vi "tool go3.vi"(4 "sensor angle":dbl=0.7625468656636853, 5 "assembly angle":dbl=0.7934896104592445, 6 "sensor center":dbl[](array[numeric])=[1019.8477869592303, 797.7567932559023], 7 "assembly center":dbl[](array[numeric])=[988.6776511594305, 1093.1610787780178], 9 "motion":T3={"XYZU "=[], "XY speed"=20.0, "Z speed"=3.0, "U speed"=0.0}, 10 "z offset":T1={"Syringe Z0"=65.0, "assembly thickness"=1.476, "tool height"=9.5, "Gule thickness "=0.1, "Pick Up Tool Z height"=63.541299073279426, "assembly Z offset"=-4.7, "gule distances"=0.6, "Syringe Z height abs"=53.424, "assembly Z height abs"=56.041299073279426, "Syringe Z height rel"=-11.576, "assembly Z height rel"=-2.8, "component  thickness"=1.224}, 11 "controller in":T4={"A3200.lvclass"=refnum, "Ultimus V2.lvclass"=refnum, "NI-DAQ.lvclass"=refnum, "Motion.lvclass"=refnum, "I-O.lvclass"=refnum, "Dispenser.lvclass"=refnum}) -> (2 "z offset out":T1={"Syringe Z0"=65.0, "assembly thickness"=1.476, "tool height"=9.5, "Gule thickness "=0.1, "Pick Up Tool Z height"=63.541299073279426, "assembly Z offset"=-4.7, "gule distances"=0.6, "Syringe Z height abs"=53.424, "assembly Z height abs"=56.041299073279426, "Syringe Z height rel"=-11.576, "assembly Z height rel"=-2.8, "component  thickness"=1.224}, 3 "controller out":T4)   [LabVIEW 2016]
uses:
  Classes/Controller/Motion/A3200 Folder/A3200.lvclass
  D:/Gantry_General/Classes/Controller/Motion/Motion Folder/Motion.lvclass
  Classes/Controller/Dispenser/Ultimus V2 Folder/Ultimus V2.lvclass
  Classes/Controller/I-O/NI-DAQ Folder/NI-DAQ.lvclass
  D:/Gantry_General/Classes/Controller/I-O/I-O Folder/I-O.lvclass
  Classes/Controller/Motion/Motion Folder/Motion.lvclass
  Classes/Controller/I-O/I-O Folder/I-O.lvclass
  Classes/Controller/Dispenser/Dispenser Folder/Dispenser.lvclass
panel:
  in  "run 2":bool
  in  "run":bool
  in  "Tab Control":T2(tab)=enum."motion"
  in  "go to assembly xyzu":bool
  in  "get assembly xyzu":bool
  out "assembly xyzu":dbl[](array[numeric])=[868.8146511594305, 1082.6710787780178, 56.041299073279426, 0.03094274479555914]
  in  "go to assembly center":bool
  in  "get assembly center":bool
  in  "go to tool center":bool
  in  "go to sensor center":bool
  in  "Bellows tool offset":dbl[](array[numeric])=[-119.863, -10.49, 0.0, 0.0]
  in  "get tool center":bool
  in  "tooling center":dbl[](array[numeric])=[1209.998534492856, 792.2969774938225]
  in  "get sensor center":bool
  in  "tooling angle":dbl=0.0876326779785796
  in  "Speed":dbl=30.0
  in  "Delay Time (s)":dbl=10.0
  out "angle":dbl=1.772888683335932
  in  "assembly z":dbl=57.43
  in  "get tooling xyzu":bool
  out "tooling center xyzu":dbl[](array[numeric])=[1090.1355344928559, 781.8069774938225, 0.0, 0.0]
  in  "go to tooling center xyzu":bool
  in  "z go":bool
  out "Sum":dbl[](array[numeric])=[1219.30639899585, 722.8896830877354, 52.864847366341415, 0.003106741190800654] format="%#_8g"
  in  "joystick and camera":bool
  in  "set z height":bool
  out "XYZTheta Out":dbl[](array[numeric])=[1090.1355359956099, 781.8069698988636, 63.541299073279426, 9.091827430758793e-07]
  in  "z to zero":bool
  in  "go to Lower stop":bool
  out "Boolean":bool
  in  "Position":dbl format="%#_13g"
  in  "IO 1":bool
  in  "IO 2":bool
  in  "Values":bool[](array[boolean])=[FALSE, FALSE]
  in  "Indices":i32[](array[numeric])=[0, 20]
  in  "Value":bool
  in  "Channel":i32
  out "Array 2":bool[](array[boolean])
  out "Value 2":bool
  in  "stop":bool
  # "57.53"
  # "57.21"
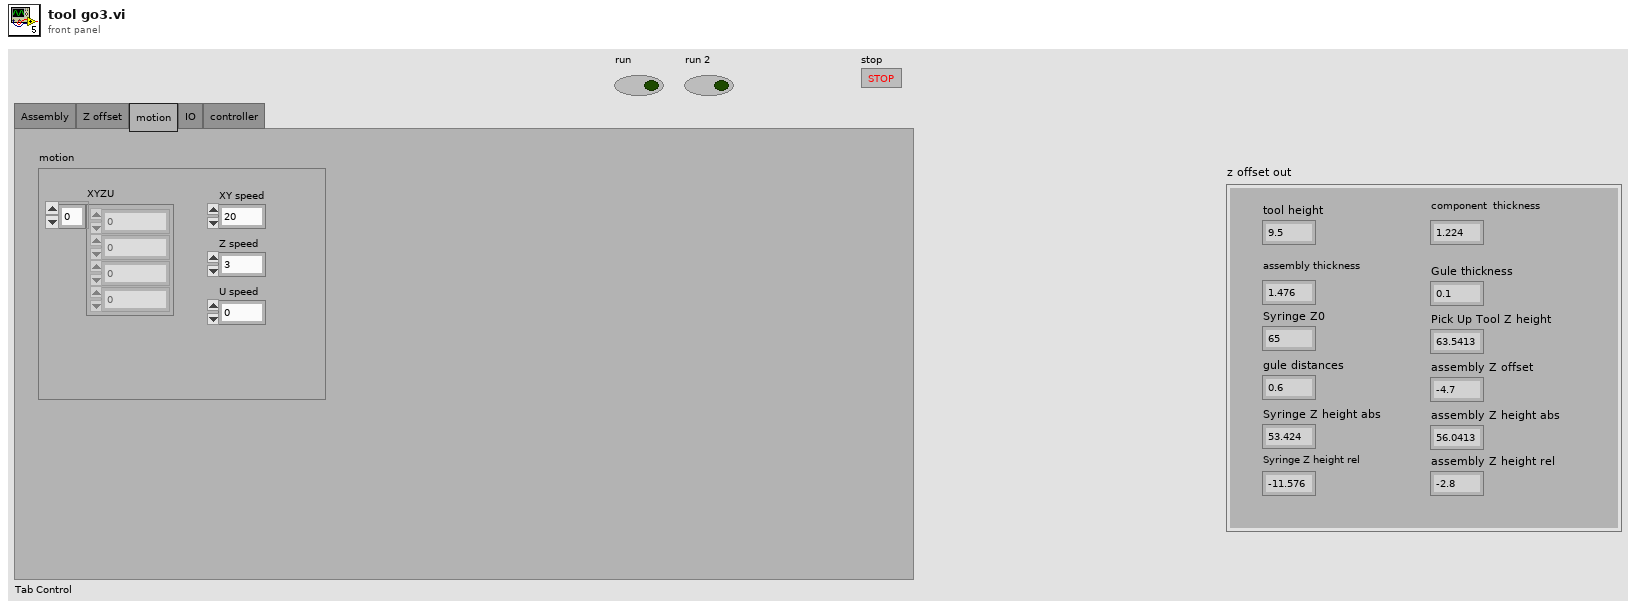
[diagram p1: front panel]
types:
  T1 = cluster{"Syringe Z0":dbl, "assembly thickness":dbl, "tool height":dbl, "Gule thickness ":dbl, "Pick Up Tool Z height":dbl, "assembly Z offset":dbl, "gule distances":dbl, "Syringe Z height abs":dbl, "assembly Z height abs":dbl, "Syringe Z height rel":dbl, "assembly Z height rel":dbl, "component  thickness":dbl}
  T2 = enum32{"Assembly", "Z offset", "motion", "IO", "controller"}
  T3 = cluster{"XYZU ":dbl[], "XY speed":dbl, "Z speed":dbl, "U speed":dbl}
  T4 = cluster{"A3200.lvclass":refnum<class "A3200.lvclass">, "Ultimus V2.lvclass":refnum<class "Ultimus V2.lvclass">, "NI-DAQ.lvclass":refnum<class "NI-DAQ.lvclass">, "Motion.lvclass":refnum<class "Motion.lvclass">, "I-O.lvclass":refnum<class "I-O.lvclass">, "Dispenser.lvclass":refnum<class "Dispenser.lvclass">}
  T5 = cluster{"Bellows tool offset":dbl[], "tooling center":dbl[], "tooling angle ":dbl, "sensor center":dbl[], "sensor angle":dbl, "assembly center":dbl[], "assembly angle":dbl}
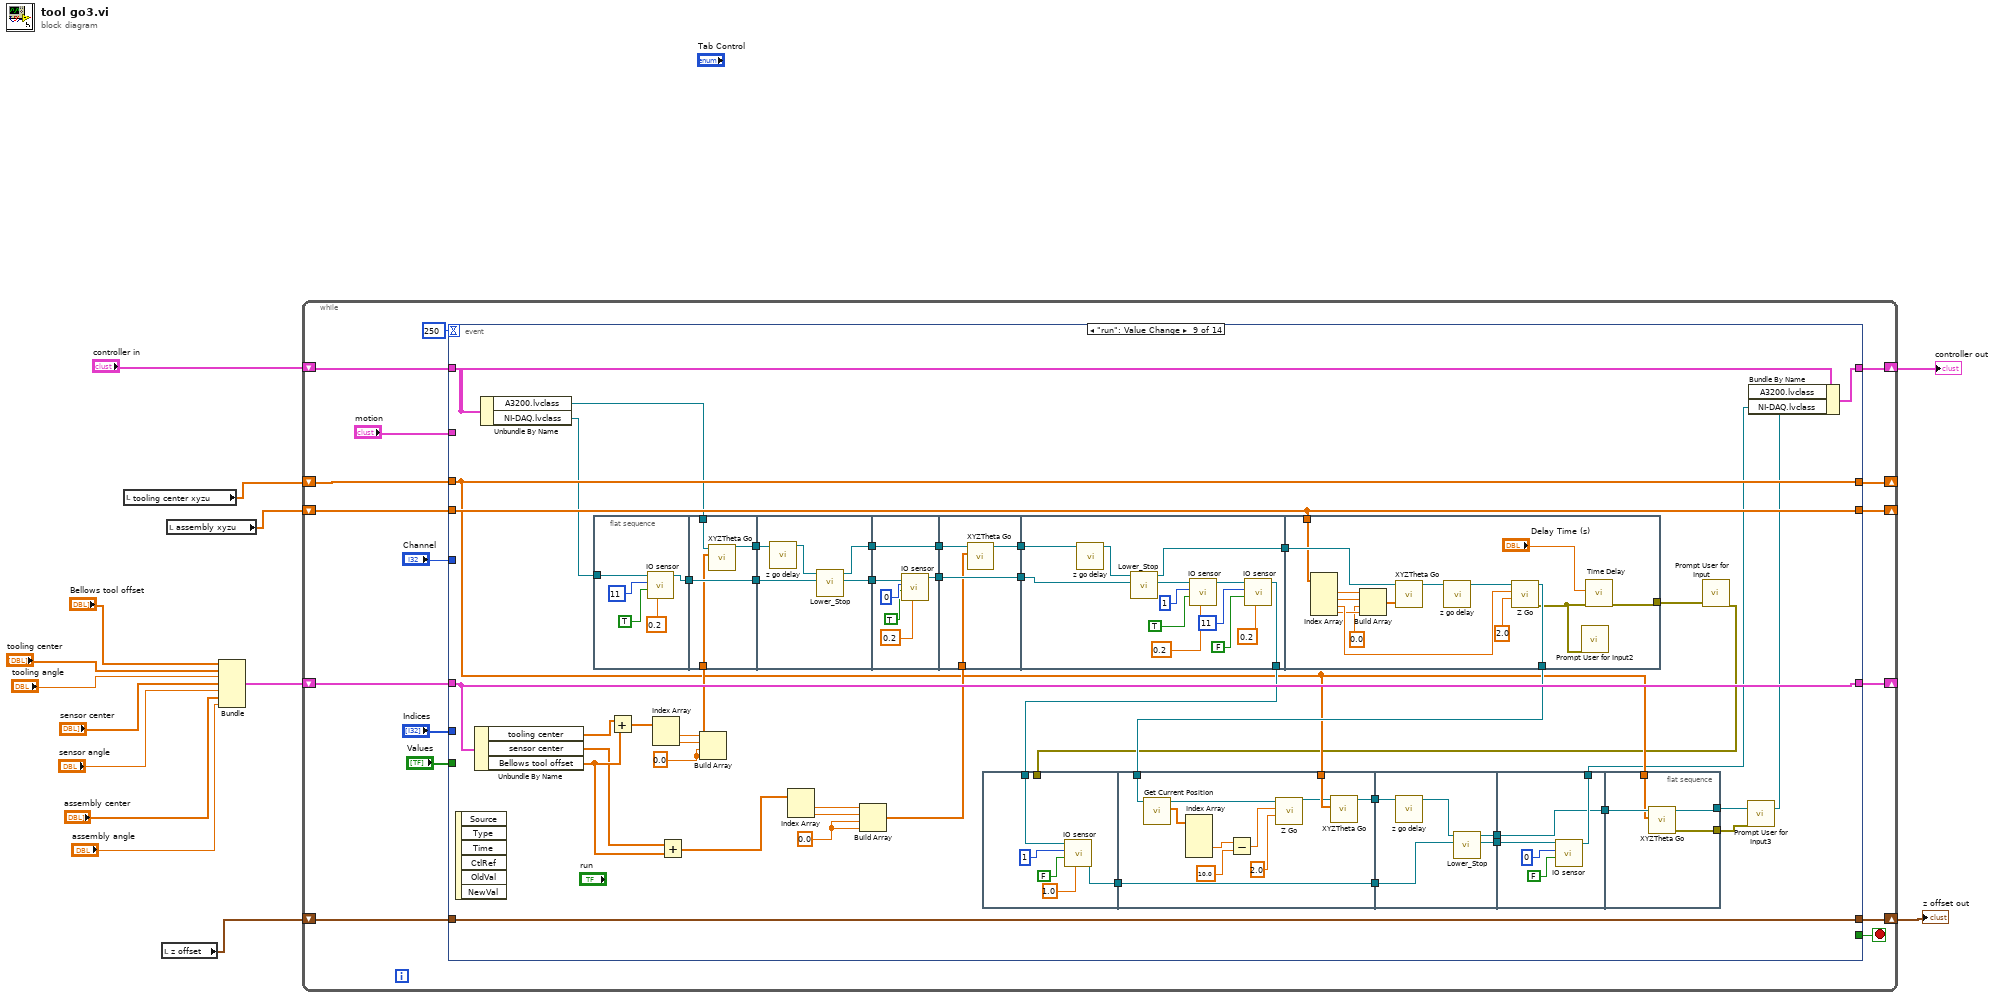
[diagram p0: block diagram]
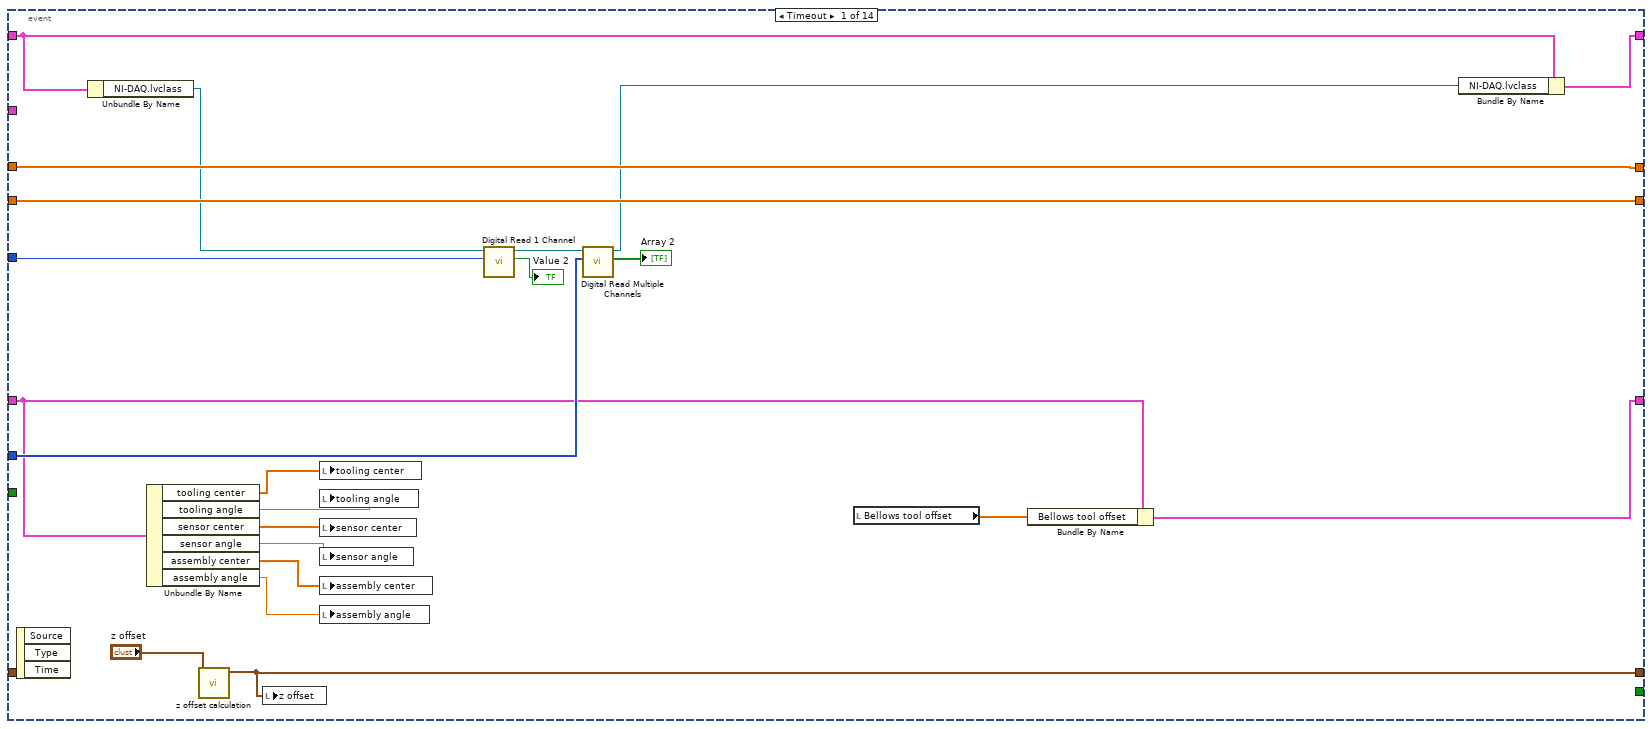
[diagram p2: hidden frame]
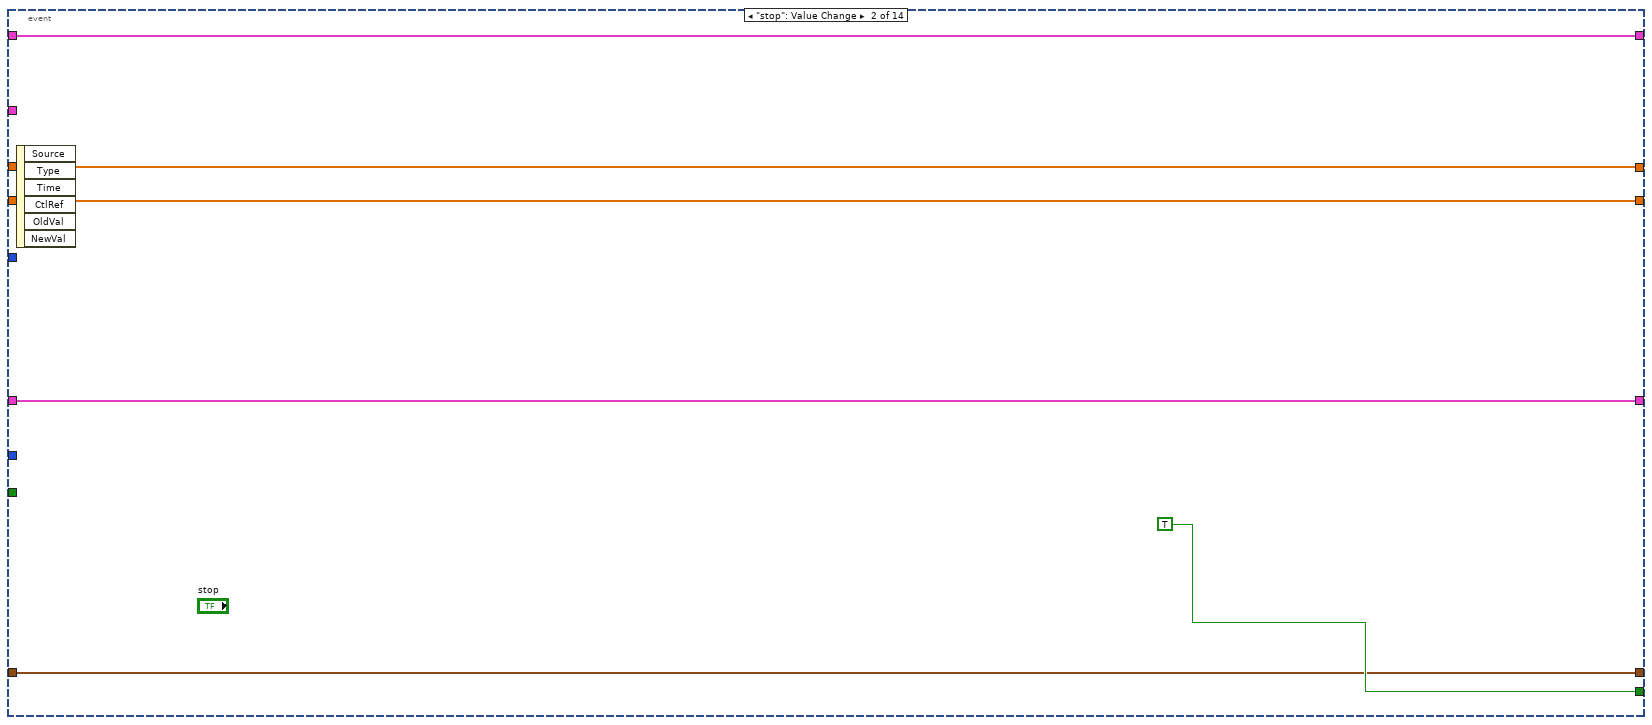
[diagram p3: hidden frame]
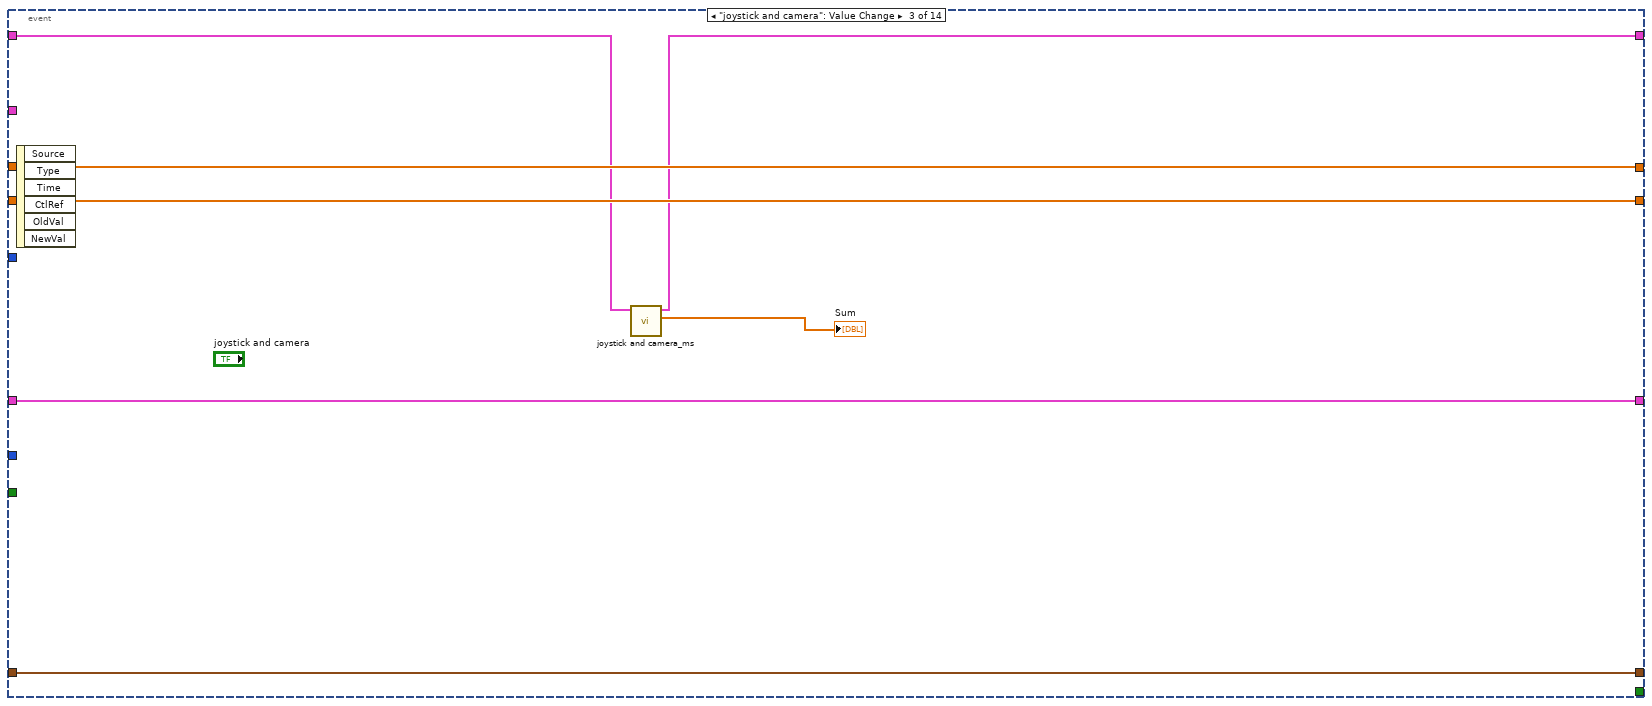
[diagram p4: hidden frame]
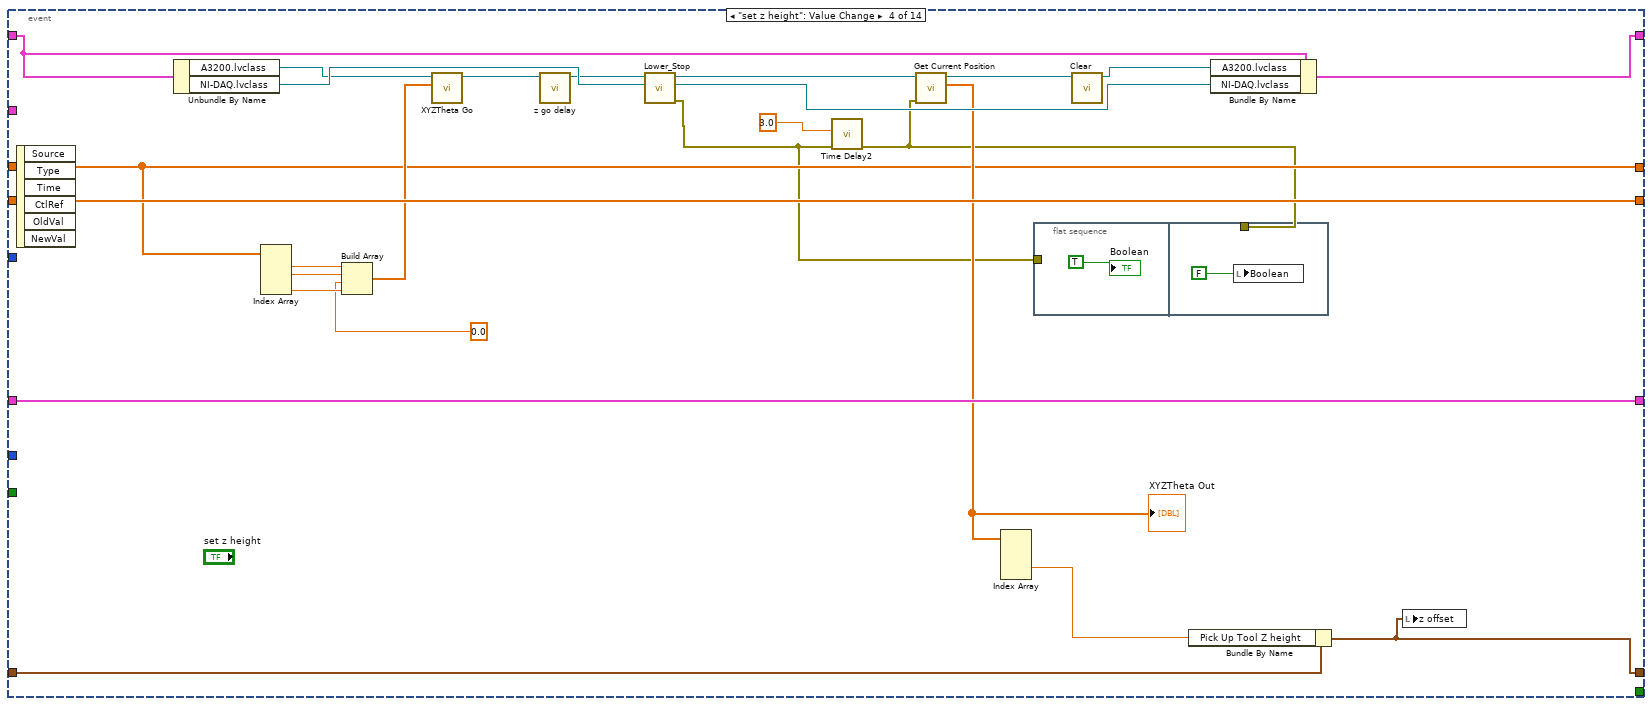
[diagram p5: hidden frame]
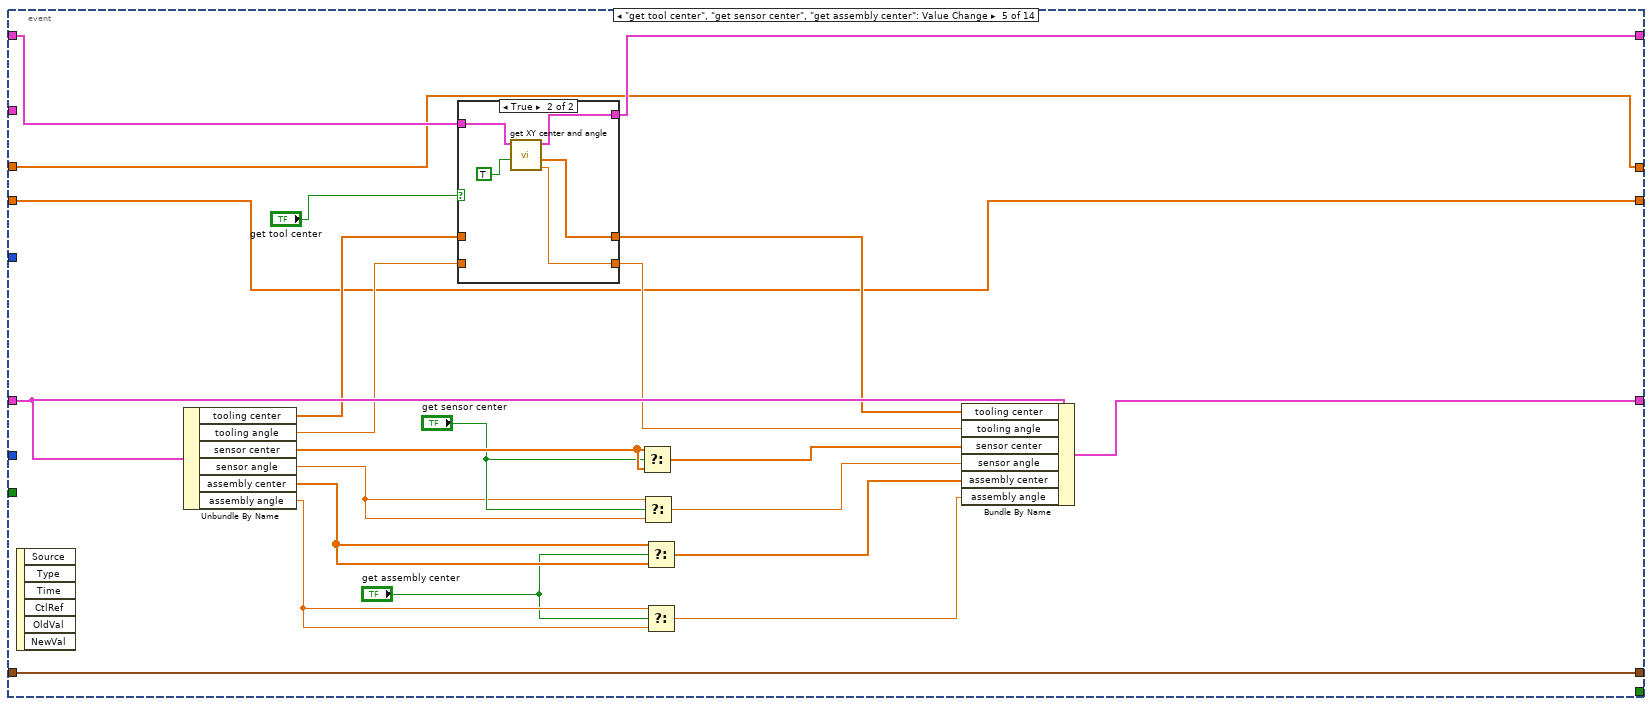
[diagram p6: hidden frame]
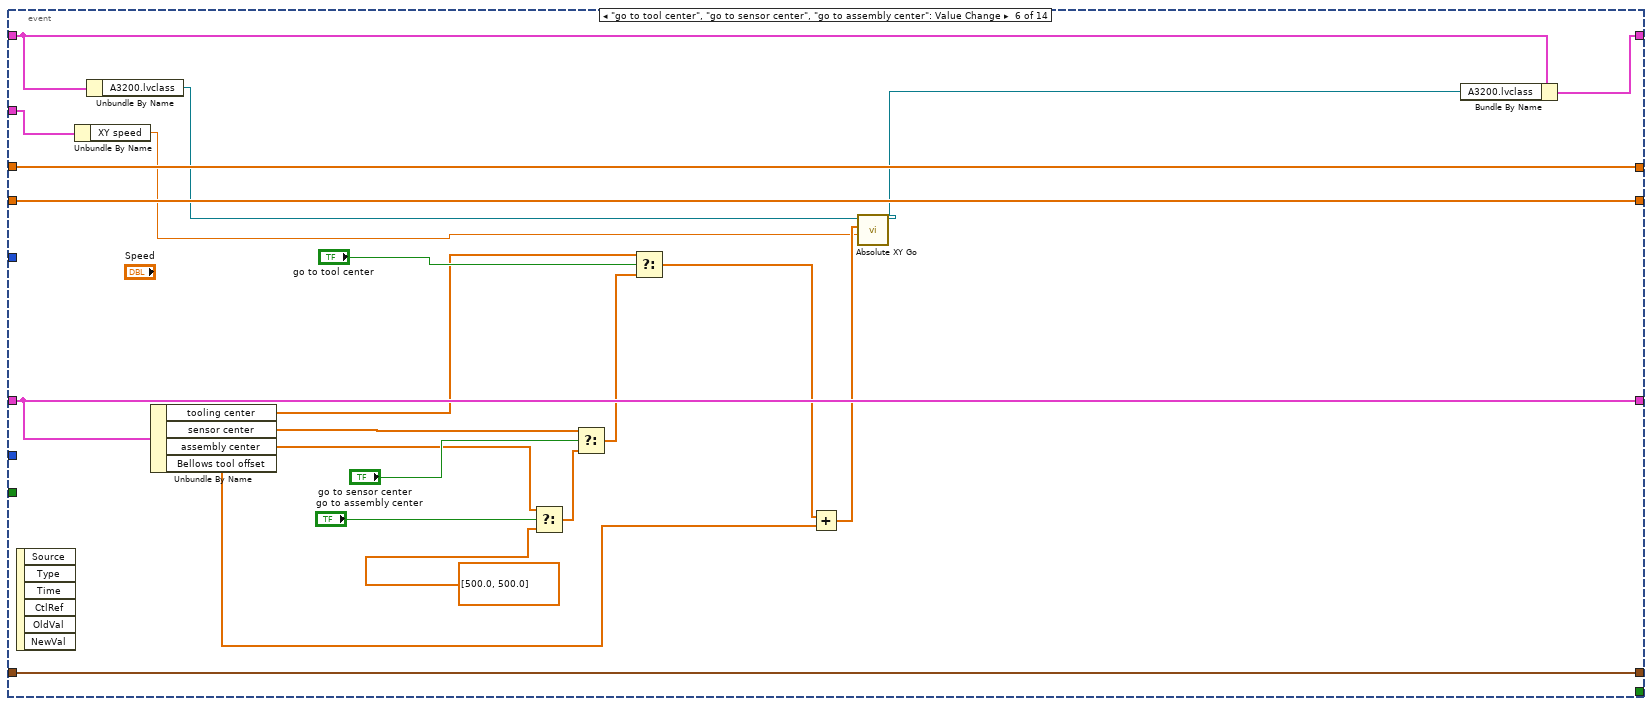
[diagram p8: hidden frame]
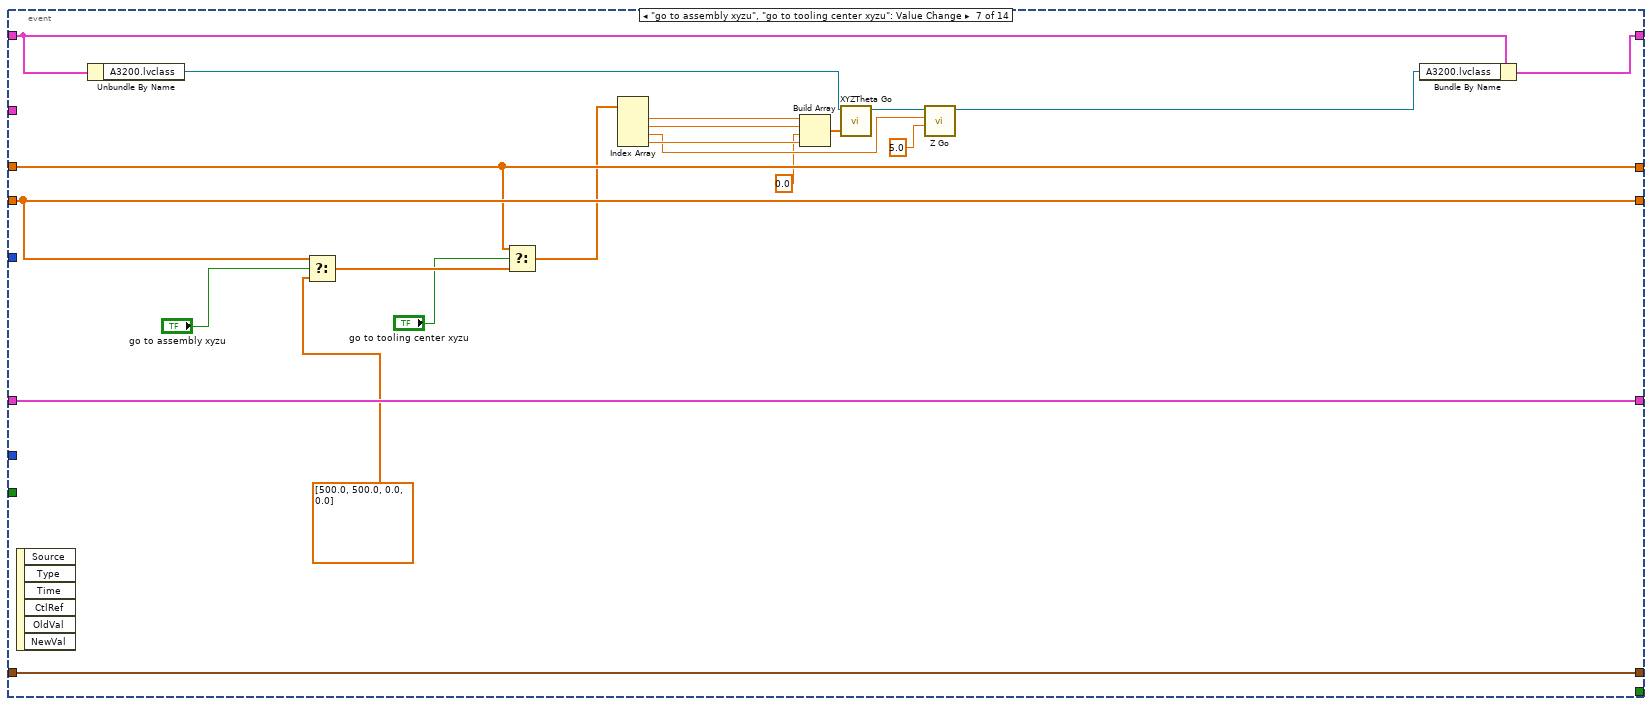
[diagram p9: hidden frame]
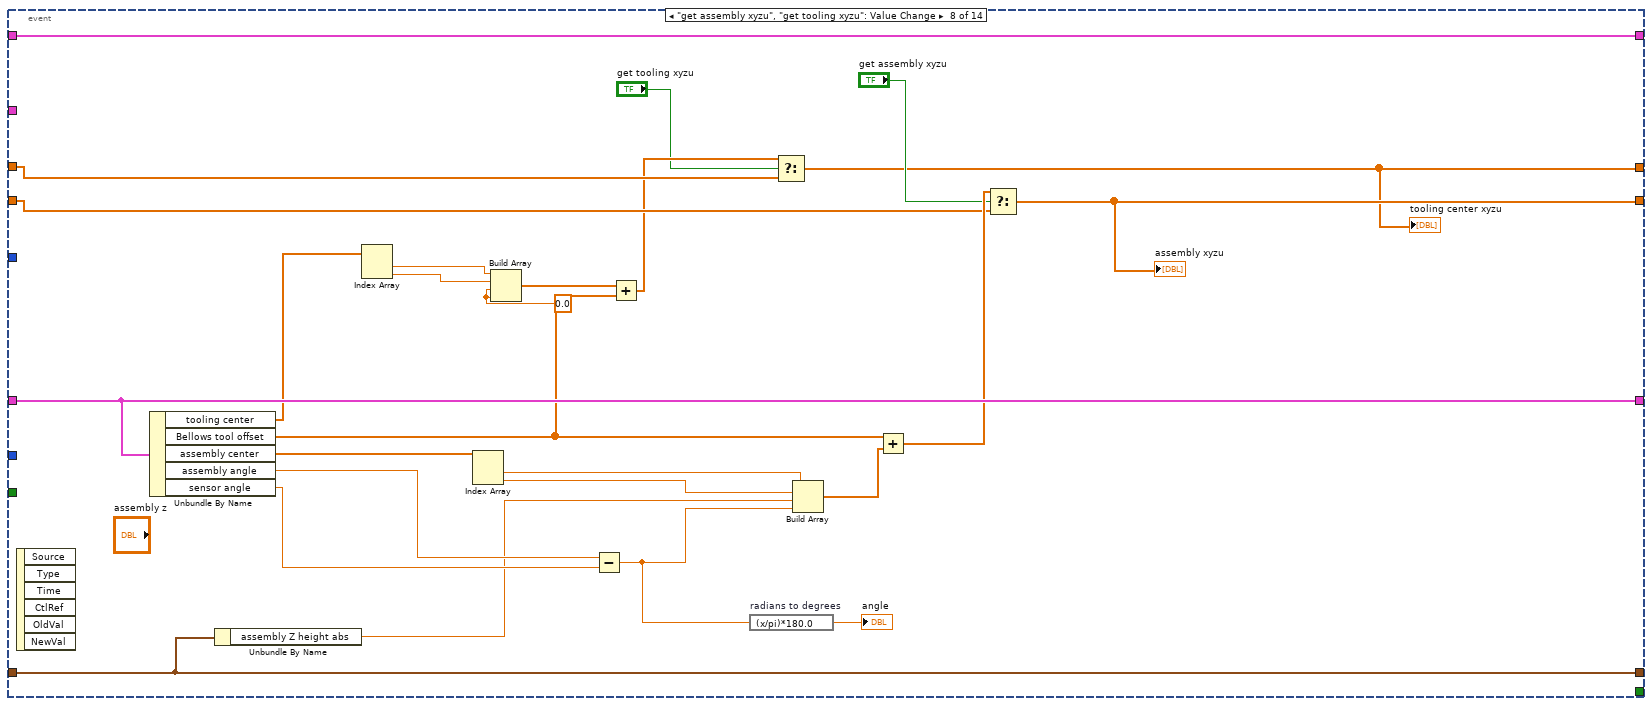
[diagram p10: hidden frame]
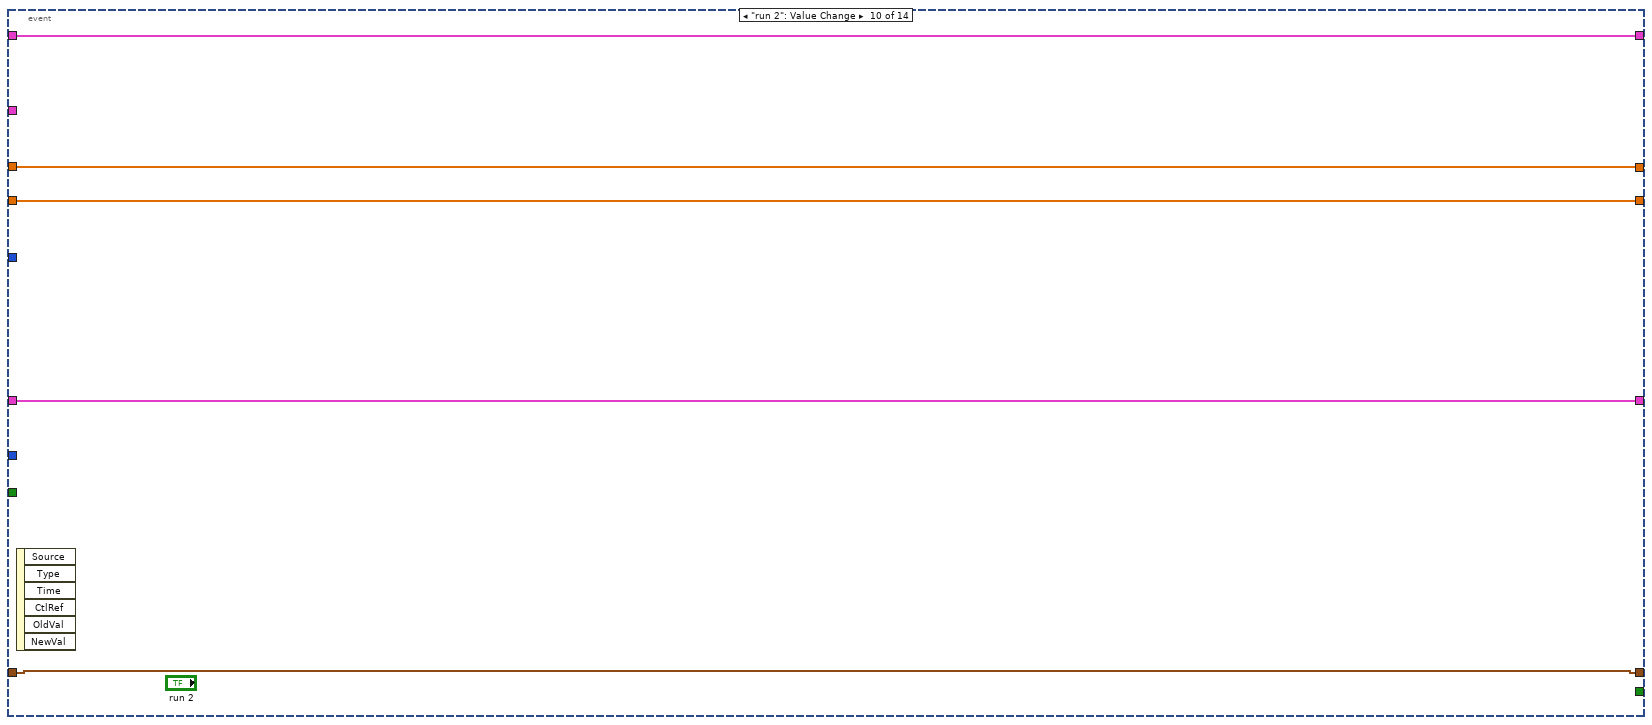
[diagram p11: hidden frame]
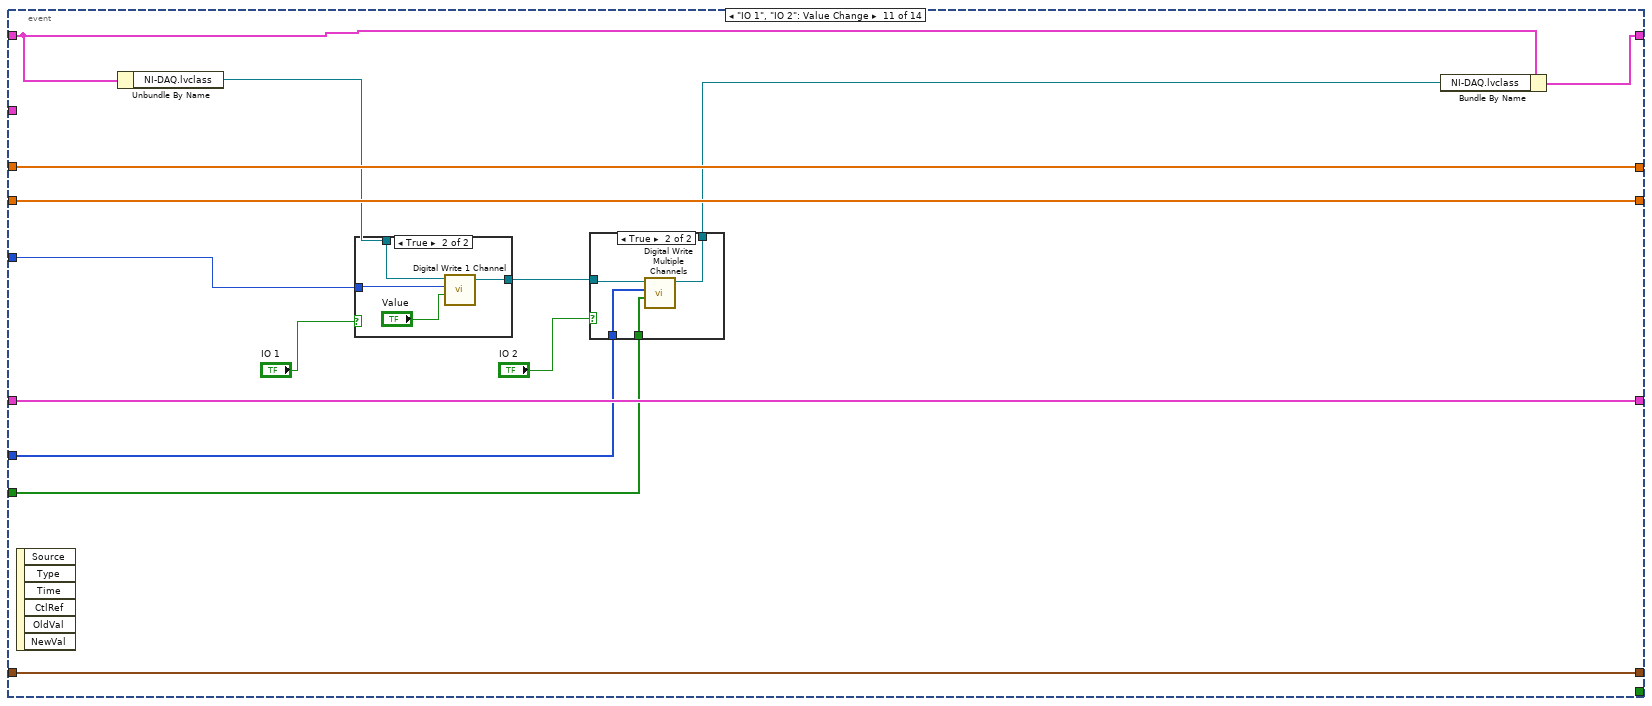
[diagram p12: hidden frame]
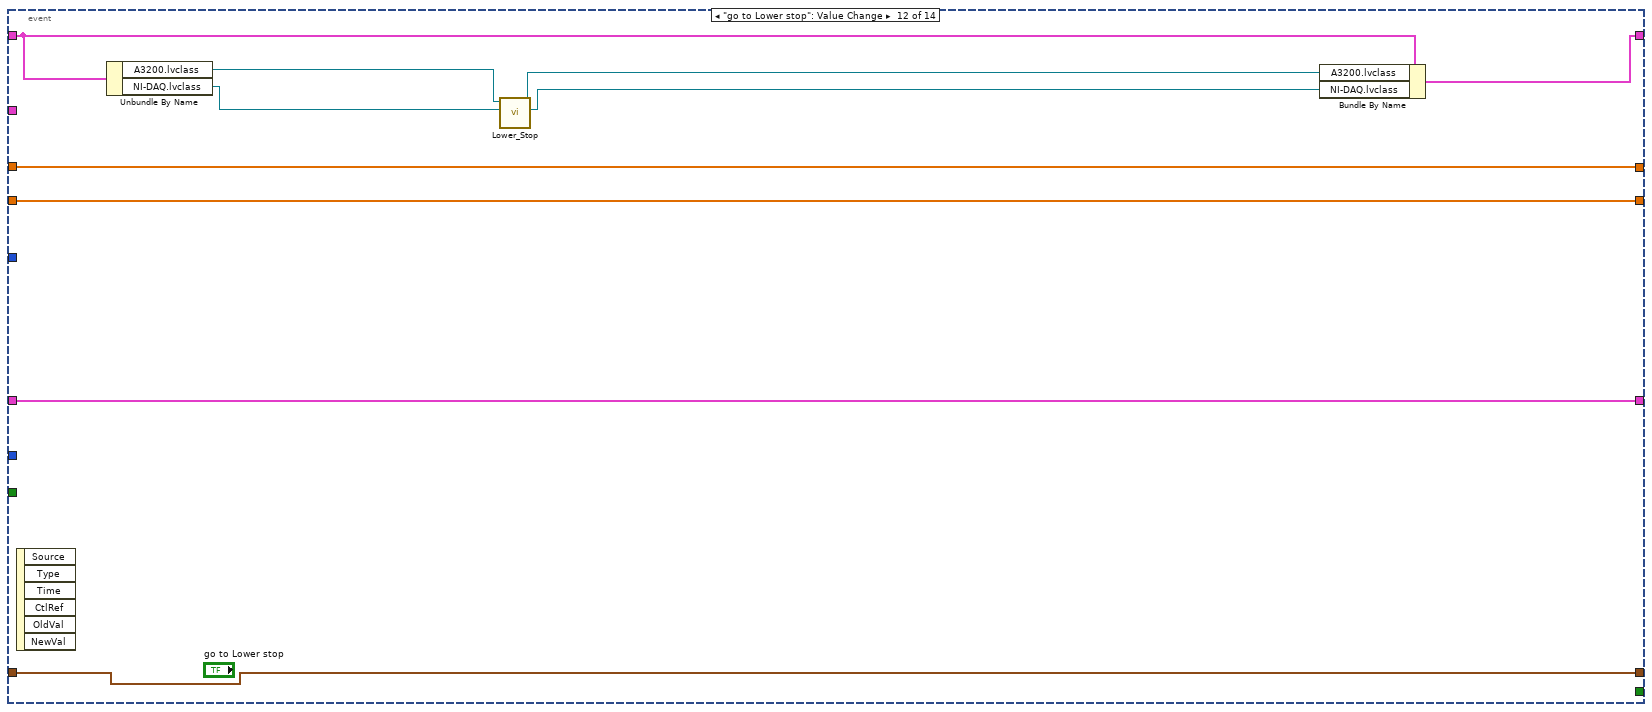
[diagram p15: hidden frame]
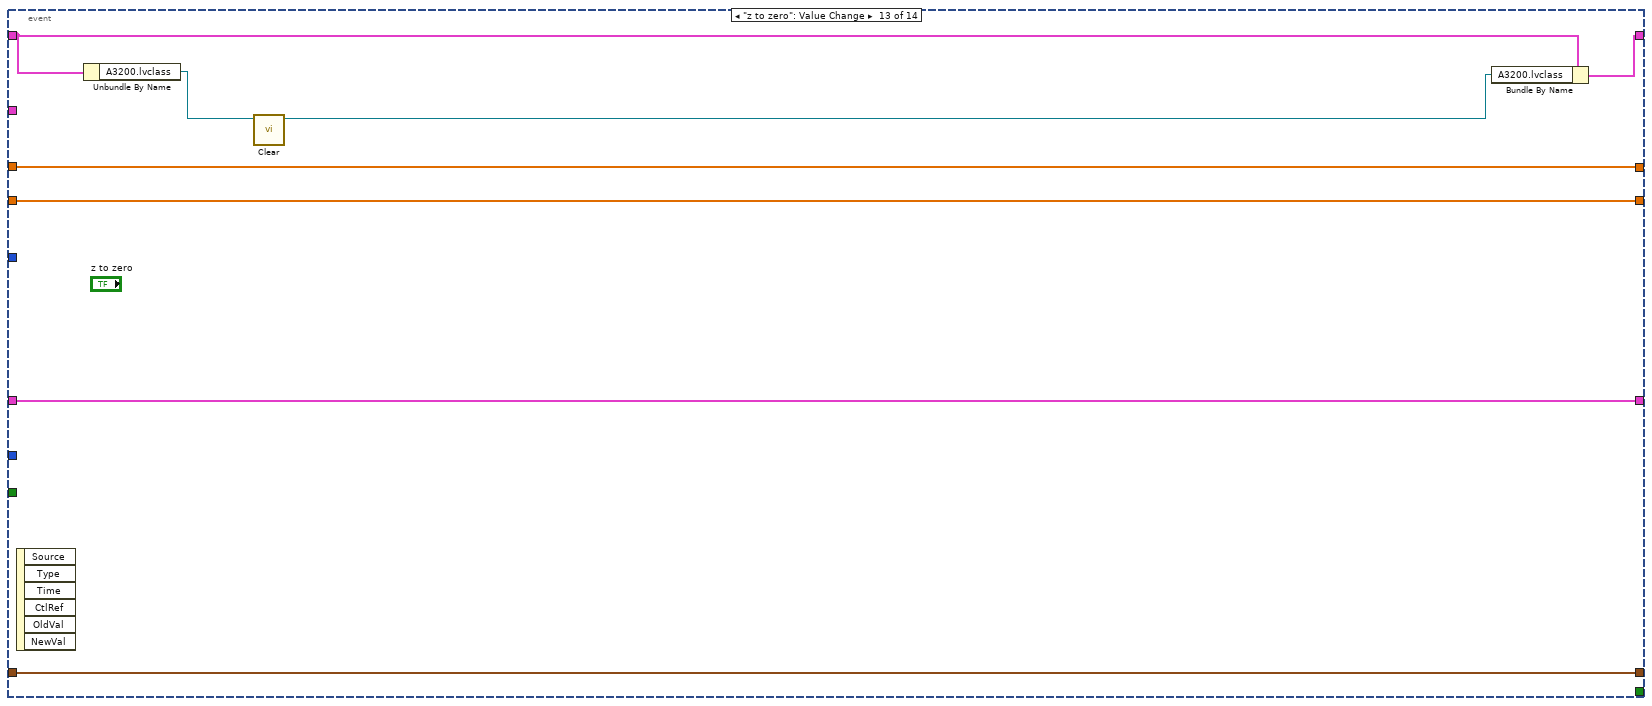
[diagram p16: hidden frame]
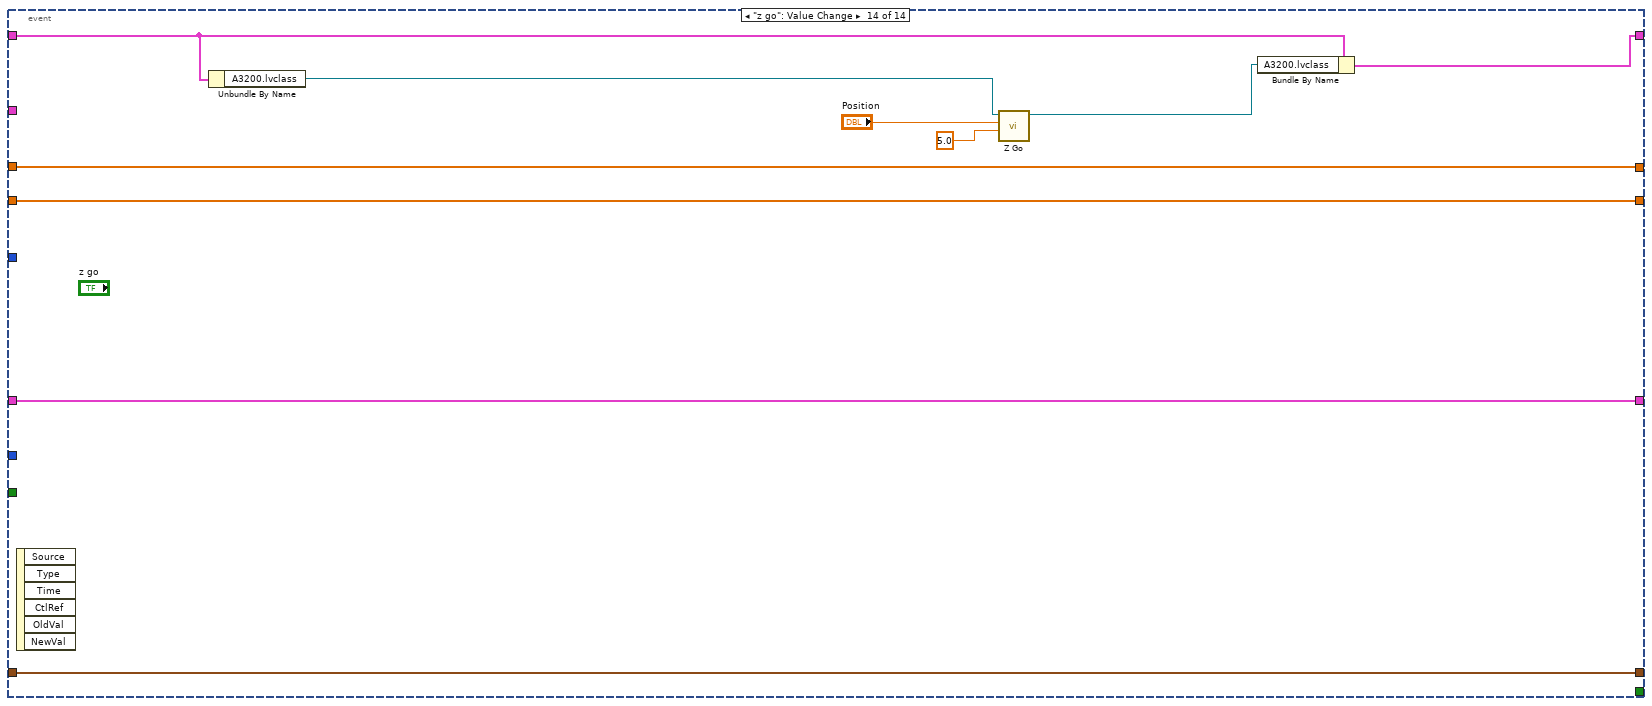
[diagram p17: hidden frame]
diagram:
  n1 = local read "tooling center xyzu"() -> (w6:dbl[])
  n2 = local read "z offset"() -> (w2:T1)
  n3 = local read "assembly xyzu"() -> (w5:dbl[])
  n4 = Bundle("Bellows tool offset"="Bellows tool offset", "tooling center"="tooling center", "tooling angle"="tooling angle", "sensor center"="sensor center", "sensor angle"="sensor angle", "assembly center"="assembly center", "assembly angle"="assembly angle") -> (w8:T5)  [unwired: 1 in]
  n5 = while {
    shift-right: [w27] -> _
    shift-left: w8 -> [w28]
    shift-right: [w25] -> _
    shift-left: w5 -> [w21]
    shift-right: [w19] -> _
    shift-left: w6 -> [w20]
    shift-right: [w18] -> w3
    shift-left: "controller in" -> [w26]
    shift-right: [w16] -> w1
    shift-left: w2 -> [w17]
    stop <- w30 stop-if-true
    n6 = event shown="[8] \"run\": Value Change" {
      selector: _ -> [_ _ _ _ _ _ _ _ _ _ _ _ _ _]
      dyn-events: _ -> [_ _ _ _ _ _ _ _ _ _ _ _ _ _]
      timeout: 250 -> [_ _ _ _ _ _ _ _ _ _ _ _ _ _]
      tunnel: [_ TRUE _ _ _ _ _ _ _ _ _ _ _ _] -> w30
      tunnel: [w45 w57 w65 w90 w114 w144 w165 w190 w229 w322 w336 w356 w364 w374] -> w27
      tunnel: w28 -> [w46 w57 w65 w90 w113 w144 w165 w190 w229 w322 w336 w356 w364 w374]
      tunnel: [w36 w56 w60 w82 w110 w129 w146 w191 w199 w319 w327 w353 w361 w366] -> w18
      tunnel: w26 -> [w35 w56 w61 w83 w109 w127 w148 w191 w200 w319 w325 w352 w359 w367]
      tunnel: w21 -> [w52 w55 w64 w89 w96 w134 w162 w177 w223 w321 w335 w355 w363 w373]
      tunnel: [w52 w55 w64 w89 w96 w134 w162 w169 w223 w321 w335 w355 w363 w373] -> w25
      tunnel: "Channel" -> [w50 _ _ _ _ _ _ _ _ _ w332 _ _ _]
      tunnel: "Values" -> [_ _ _ _ _ _ _ _ _ _ w331 _ _ _]
      tunnel: "Indices" -> [w49 _ _ _ _ _ _ _ _ _ w330 _ _ _]
      tunnel: w20 -> [w37 w54 w63 w74 w94 w130 w161 w175 w201 w320 w328 w354 w362 w372]
      tunnel: [w37 w54 w63 w74 w94 w130 w161 w168 w201 w320 w328 w354 w362 w372] -> w19
      tunnel: w17 -> [_ w53 w62 w81 w93 w125 w145 w167 w194 w318 w323 w347 w357 w371]
      tunnel: [w32 w53 w62 w69 w93 w125 w145 w167 w194 w318 w323 w347 w357 w371] -> w16
      tunnel: "motion" -> [_ _ _ _ _ w124 _ _ _ _ _ _ _ _]
      event Timeout {
        n7 = event-data() -> ()  [unwired: 1 in, 3 out]
        n8 = Unbundle By Name(w35) -> ("NI-DAQ.lvclass"=w33:refnum<class "NI-DAQ.lvclass">)
        n9 = Unbundle By Name(w46) -> ("tooling center"=w38:dbl[], "tooling angle"=w43:dbl, "sensor center"=w42:dbl[], "sensor angle"=w41:dbl, "assembly center"=w40:dbl[], "assembly angle"=w39:dbl)
        n10 = call "z offset calculation.vi"("z offset in"="z offset") -> ("z offset out"=w32:T1)  [unwired: 10 in]
        n11 = local write "z offset"(w32) -> ()
        n12 = local write "tooling center"(w38) -> ()
        n13 = local write "tooling angle"(w43) -> ()
        n14 = local write "sensor center"(w42) -> ()
        n15 = local write "sensor angle"(w41) -> ()
        n16 = local write "assembly center"(w40) -> ()
        n17 = local write "assembly angle"(w39) -> ()
        n18 = call-dynamic "Digital Read 1 Channel.vi"("Read"=w50, "NI-DAQ in"=w33) -> ("Value"=→"Value 2":bool, "NI-DAQ out"=w51:refnum<class "NI-DAQ.lvclass">)  [unwired: 7 in, 1 out]
        n19 = call-dynamic "Digital Read Multiple Channels.vi"("Array"=w49, "NI-DAQ in"=w51) -> ("subarray"=→"Array 2":bool[], "NI-DAQ out"=w34:refnum<class "NI-DAQ.lvclass">)  [unwired: 7 in, 1 out]
        n20 = local read "Bellows tool offset"() -> (w44:dbl[])
        n21 = Bundle By Name(cluster=w46, "Bellows tool offset"=w44) -> (w45:T5)
        n22 = Bundle By Name(cluster=w35, "NI-DAQ.lvclass"=w34) -> (w36:T4)
      }
      event "stop": Value Change {
        n23 = event-data() -> ()  [unwired: 1 in, 6 out]
      }
      event "joystick and camera": Value Change {
        n24 = event-data() -> ()  [unwired: 1 in, 6 out]
        n25 = call "joystick and camera_ms.vi"("controller in"=w61) -> ("Gantry"=→"Sum":dbl[], "controller out"=w60:T4)  [unwired: 9 in]
      }
      event "set z height": Value Change {
        n26 = event-data() -> ()  [unwired: 1 in, 6 out]
        n27 = Unbundle By Name(w83) -> ("A3200.lvclass"=w75:refnum<class "A3200.lvclass">, "NI-DAQ.lvclass"=w88:refnum<class "NI-DAQ.lvclass">)
        n28 = Index Array(array=w74) -> (element #1=w79:dbl, element #2=w78:dbl, element #4=w77:dbl)  [unwired: 4 in, 1 out]
        n29 = Build Array(w79, w78, 0.0 ("element"), w77) -> (w80:dbl[])
        n30 = call "XYZTheta Go.vi"("XYZTheta In"=w80, "Motion in"=w75) -> ("Motion out"=w66:refnum<class "A3200.lvclass">)  [unwired: 7 in, 2 out]
        n31 = call "z go delay.vi"("Motion.lvclass"=w66) -> ("Motion.lvclass 2"=w67:refnum<class "A3200.lvclass">)  [unwired: 10 in]
        n32 = call "Lower_Stop.vi"("I-O in"=w88, "Motion in"=w67) -> ("error out"=w70:errorcluster, "I-O out"=w87:refnum<class "NI-DAQ.lvclass">, "Motion out"=w86:refnum<class "A3200.lvclass">)  [unwired: 7 in]
        n33 = call "Time Delay2"("error in (no error)"=w70, "Delay Time (s)"=3.0) -> ("error out"=w68:errorcluster)  [unwired: 9 in]
        n34 = call-dynamic "Get Current Position.vi"("error in (no error)"=w68, "Gantry in"=w86) -> ("XYZTheta Out"=w85:dbl[], "Gantry out"=w73:refnum<class "A3200.lvclass">)  [unwired: 7 in, 1 out]
        "XYZTheta Out" <- w85
        n35 = Index Array(array=w85) -> (element #3=w84:dbl)  [unwired: 4 in, 3 out]
        n36 = flat-sequence {
          tunnel: w70 -> [_]
          tunnel: w68 -> [_]
          frame #0 {
            "Boolean" <- TRUE
          }
          frame #1 {
            n37 = local write "Boolean"(FALSE) -> ()
          }
        }
        n38 = call "Clear.vi"("Motion in"=w73) -> ("Motion out"=w72:refnum<class "A3200.lvclass">)  [unwired: 9 in, 1 out]
        n39 = Bundle By Name(cluster=w81, "Pick Up Tool Z height"=w84) -> (w69:T1)
        n40 = Bundle By Name(cluster=w83, "A3200.lvclass"=w72, "NI-DAQ.lvclass"=w87) -> (w82:T4)
        n41 = local write "z offset"(w69) -> ()
      }
      event "get tool center", "get sensor center", "get assembly center": Value Change {
        n42 = event-data() -> ()  [unwired: 1 in, 6 out]
        n43 = Unbundle By Name(w113) -> ("tooling center"=w105:dbl[], "tooling angle"=w104:dbl, "sensor center"=w102:dbl[], "sensor angle"=w100:dbl, "assembly center"=w111:dbl[], "assembly angle"=w112:dbl)
        n44 = case shown="True" "get tool center" {
          tunnel: [w117 w119] -> w110
          tunnel: w109 -> [w117 w118]
          tunnel: [w116 w122] -> w107
          tunnel: [w115 w121] -> w106
          tunnel: w105 -> [w116 _]
          tunnel: w104 -> [w115 _]
          frame False {
          }
          frame True {
            n45 = call "get XY center and angle.vi"("output P1 XY"=TRUE, "controller in"=w118) -> ("XY theta out"=w121:dbl, "XY center out"=w122:dbl[], "controller out"=w119:T4)  [unwired: 6 in, 1 out]
          }
        }
        n46 = Select(t=w102, s="get sensor center", f=w102) -> (s? t:f=w97:dbl[])
        n47 = Select(t=w100, s="get sensor center", f=w100) -> (s? t:f=w98:dbl)
        n48 = Select(t=w111, s="get assembly center", f=w111) -> (s? t:f=w99:dbl[])
        n49 = Select(t=w112, s="get assembly center", f=w112) -> (s? t:f=w95:dbl)
        n50 = Bundle By Name(cluster=w113, "tooling center"=w107, "tooling angle"=w106, "sensor center"=w97, "sensor angle"=w98, "assembly center"=w99, "assembly angle"=w95) -> (w114:T5)
      }
      event "go to tool center", "go to sensor center", "go to assembly center": Value Change {
        n51 = event-data() -> ()  [unwired: 1 in, 6 out]
        n52 = Unbundle By Name(w124) -> ("XY speed"=w123:dbl)
        n53 = Unbundle By Name(w127) -> ("A3200.lvclass"=w126:refnum<class "A3200.lvclass">)
        n54 = Unbundle By Name(w144) -> ("tooling center"=w142:dbl[], "sensor center"=w140:dbl[], "assembly center"=w137:dbl[], "Bellows tool offset"=w131:dbl[])
        n55 = Select(t=w137, s="go to assembly center", f=dbl[] [500.0, 500.0]) -> (s? t:f=w138:dbl[])
        n56 = Select(t=w140, s="go to sensor center", f=w138) -> (s? t:f=w141:dbl[])
        n57 = Select(t=w142, s="go to tool center", f=w141) -> (s? t:f=w132:dbl[])
        n58 = Add(x=w132, y=w131) -> (x+y=w133:dbl[])
        n59 = call-dynamic "Absolute XY Go.vi"("Speed"=w123, "XY"=w133, "Gantry in"=w126) -> ("Gantry out"=w128:refnum<class "A3200.lvclass">)  [unwired: 7 in, 1 out]
        n60 = Bundle By Name(cluster=w127, "A3200.lvclass"=w128) -> (w129:T4)
      }
      event "go to assembly xyzu", "go to tooling center xyzu": Value Change {
        n61 = event-data() -> ()  [unwired: 1 in, 6 out]
        n62 = Unbundle By Name(w148) -> ("A3200.lvclass"=w149:refnum<class "A3200.lvclass">)
        n63 = Select(t=w162, s="go to assembly xyzu", f=dbl[] [500.0, 500.0, 0.0, 0.0]) -> (s? t:f=w163:dbl[])
        n64 = Select(t=w161, s="go to tooling center xyzu", f=w163) -> (s? t:f=w153:dbl[])
        n65 = Index Array(array=w153) -> (element #1=w157:dbl, element #2=w156:dbl, element #3=w152:dbl, element #4=w155:dbl)  [unwired: 4 in]
        n66 = Build Array(w157, w156, 0.0 ("element"), w155) -> (w158:dbl[])
        n67 = call "XYZTheta Go.vi"("XYZTheta In"=w158, "Motion in"=w149) -> ("Motion out"=w151:refnum<class "A3200.lvclass">)  [unwired: 7 in, 2 out]
        n68 = call-dynamic "Z Go.vi"("Speed"=5.0, "Position"=w152, "Gantry in"=w151) -> ("Gantry out"=w147:refnum<class "A3200.lvclass">)  [unwired: 7 in, 1 out]
        n69 = Bundle By Name(cluster=w148, "A3200.lvclass"=w147) -> (w146:T4)
      }
      event "get assembly xyzu", "get tooling xyzu": Value Change {
        w185 = 0.0 ("element")
        n70 = event-data() -> ()  [unwired: 1 in, 6 out]
        n71 = Unbundle By Name(w190) -> ("tooling center"=w183:dbl[], "Bellows tool offset"=w180:dbl[], "assembly center"=w189:dbl[], "assembly angle"=w186:dbl, "sensor angle"=w172:dbl)
        n72 = Unbundle By Name(w167) -> ("assembly Z height abs"=w166:dbl)
        n73 = Index Array(array=w183) -> (element #1=w182:dbl, element #2=w181:dbl)  [unwired: 2 in]
        n74 = Index Array(array=w189) -> (element #1=w188:dbl, element #2=w187:dbl)  [unwired: 2 in]
        n75 = Build Array(w182, w181, w185, w185) -> (w179:dbl[])
        n76 = Subtract(x=w186, y=w172) -> (x-y=w171:dbl)
        n77 = Add(x=w179, y=w180) -> (x+y=w174:dbl[])
        n78 = expression code="(x/pi)*180.0" "radians to degrees"(w171) -> (→"angle":dbl)
        n79 = Select(t=w174, s="get tooling xyzu", f=w175) -> (s? t:f=w168:dbl[])
        "tooling center xyzu" <- w168
        n80 = Build Array(w188, w187, w166, w171) -> (w184:dbl[])
        n81 = Add(x=w180, y=w184) -> (x+y=w178:dbl[])
        n82 = Select(t=w178, s="get assembly xyzu", f=w177) -> (s? t:f=w169:dbl[])
        "assembly xyzu" <- w169
      }
      event "run": Value Change {
        w230 = 0.0 ("element")
        w235 = 0.0 ("element")
        n83 = event-data() -> ()  [unwired: 1 in, 6 out]
        n84 = Unbundle By Name(w229) -> ("tooling center"=w227:dbl[], "sensor center"=w225:dbl[], "Bellows tool offset"=w226:dbl[])
        n85 = Unbundle By Name(w200) -> ("A3200.lvclass"=w197:refnum<class "A3200.lvclass">, "NI-DAQ.lvclass"=w198:refnum<class "NI-DAQ.lvclass">)
        n86 = flat-sequence {
          tunnel: [w268] -> w216
          tunnel: w198 -> [w266]
          tunnel: [w274] -> w220
          tunnel: w197 -> [w273]
          tunnel: [w272] -> w217
          tunnel: w216 -> [w272]
          tunnel: w212 -> [w271]
          tunnel: w220 -> [w276]
          tunnel: [w278] -> w219
          tunnel: w217 -> [w279]
          tunnel: [w277] -> w215
          tunnel: w219 -> [w283]
          tunnel: [w283] -> w218
          tunnel: w215 -> [w282]
          tunnel: [w281] -> w213
          tunnel: [w289] -> w222
          tunnel: w218 -> [w288]
          tunnel: [w287] -> w214
          tunnel: w213 -> [w287]
          tunnel: w211 -> [w286]
          tunnel: w222 -> [w290]
          tunnel: [w298] -> w221
          tunnel: w214 -> [w297]
          tunnel: [w294] -> w204
          tunnel: w223 -> [w312]
          tunnel: w221 -> [w317]
          tunnel: [w315] -> w203
          tunnel: [w305] -> w193
          frame #0 {
            n87 = call "IO sensor.vi"("Delay Time (s)"=0.2, "Value"=TRUE, "Channel"=11, "I-O in"=w266) -> ("I-O out"=w268:refnum<class "NI-DAQ.lvclass">)  [unwired: 7 in]
          }
          frame #1 {
            n88 = call "XYZTheta Go.vi"("XYZTheta In"=w271, "Motion in"=w273) -> ("Motion out"=w274:refnum<class "A3200.lvclass">)  [unwired: 7 in, 2 out]
          }
          frame #2 {
            n89 = call "z go delay.vi"("Motion.lvclass"=w276) -> ("Motion.lvclass 2"=w275:refnum<class "A3200.lvclass">)  [unwired: 10 in]
            n90 = call "Lower_Stop.vi"("I-O in"=w279, "Motion in"=w275) -> ("I-O out"=w277:refnum<class "NI-DAQ.lvclass">, "Motion out"=w278:refnum<class "A3200.lvclass">)  [unwired: 7 in, 1 out]
          }
          frame #3 {
            n91 = call "IO sensor.vi"("Delay Time (s)"=0.2, "Value"=TRUE, "Channel"=0, "I-O in"=w282) -> ("I-O out"=w281:refnum<class "NI-DAQ.lvclass">)  [unwired: 7 in]
          }
          frame #4 {
            n92 = call "XYZTheta Go.vi"("XYZTheta In"=w286, "Motion in"=w288) -> ("Motion out"=w289:refnum<class "A3200.lvclass">)  [unwired: 7 in, 2 out]
          }
          frame #5 {
            n93 = call "z go delay.vi"("Motion.lvclass"=w290) -> ("Motion.lvclass 2"=w291:refnum<class "A3200.lvclass">)  [unwired: 10 in]
            n94 = call "Lower_Stop.vi"("I-O in"=w297, "Motion in"=w291) -> ("I-O out"=w296:refnum<class "NI-DAQ.lvclass">, "Motion out"=w298:refnum<class "A3200.lvclass">)  [unwired: 7 in, 1 out]
            n95 = call "IO sensor.vi"("Delay Time (s)"=0.2, "Value"=TRUE, "Channel"=1, "I-O in"=w296) -> ("I-O out"=w295:refnum<class "NI-DAQ.lvclass">)  [unwired: 7 in]
            n96 = call "IO sensor.vi"("Delay Time (s)"=0.2, "Value"=FALSE, "Channel"=11, "I-O in"=w295) -> ("I-O out"=w294:refnum<class "NI-DAQ.lvclass">)  [unwired: 7 in]
          }
          frame #6 {
            n97 = Index Array(array=w312) -> (element #1=w311:dbl, element #2=w310:dbl, element #3=w314:dbl, element #4=w309:dbl)  [unwired: 4 in]
            n98 = Build Array(w311, w310, 0.0 ("element"), w309) -> (w313:dbl[])
            n99 = call "XYZTheta Go.vi"("XYZTheta In"=w313, "Motion in"=w317) -> ("Motion out"=w303:refnum<class "A3200.lvclass">)  [unwired: 7 in, 2 out]
            n100 = call "z go delay.vi"("Motion.lvclass"=w303) -> ("Motion.lvclass 2"=w304:refnum<class "A3200.lvclass">)  [unwired: 10 in]
            n101 = call-dynamic "Z Go.vi"("Speed"=2.0, "Position"=w314, "Gantry in"=w304) -> ("error out"=w307:errorcluster, "Gantry out"=w315:refnum<class "A3200.lvclass">)  [unwired: 7 in]
            n102 = call "Prompt User for Input2"("error in (no error)"=w307) -> ()  [unwired: 17 in, 2 out]
            n103 = call "Time Delay"("error in (no error)"=w307, "Delay Time (s)"="Delay Time (s)") -> ("error out"=w305:errorcluster)  [unwired: 9 in]
          }
        }
        n104 = Add(x=w227, y=w226) -> (x+y=w228:dbl[])
        n105 = Index Array(array=w228) -> (element #1=w233:dbl, element #2=w234:dbl)  [unwired: 2 in]
        n106 = Add(x=w225, y=w226) -> (x+y=w224:dbl[])
        n107 = Build Array(w233, w234, w235, w235) -> (w212:dbl[])
        n108 = Index Array(array=w224) -> (element #1=w231:dbl, element #2=w232:dbl)  [unwired: 2 in]
        n109 = Build Array(w231, w232, w230, w230) -> (w211:dbl[])
        n110 = flat-sequence {
          tunnel: w204 -> [w238]
          tunnel: [w237] -> w210
          tunnel: w192 -> [_]
          tunnel: w201 -> [w251]
          tunnel: [w250] -> w209
          tunnel: [w249] -> w208
          tunnel: w210 -> [w249]
          tunnel: w203 -> [w246]
          tunnel: w209 -> [w253]
          tunnel: w208 -> [w256]
          tunnel: [w255] -> w207
          tunnel: [w254] -> w206
          tunnel: w207 -> [w259]
          tunnel: [w258] -> w196
          tunnel: [w257] -> w205
          tunnel: w206 -> [w257]
          tunnel: w205 -> [w265]
          tunnel: [w264] -> w195
          tunnel: [w263] -> w202
          tunnel: w201 -> [w262]
          frame #0 {
            n111 = call "IO sensor.vi"("Delay Time (s)"=1.0, "Value"=FALSE, "Channel"=1, "I-O in"=w238) -> ("I-O out"=w237:refnum<class "NI-DAQ.lvclass">)  [unwired: 7 in]
          }
          frame #1 {
            n112 = call-dynamic "Get Current Position.vi"("Gantry in"=w246) -> ("XYZTheta Out"=w244:dbl[], "Gantry out"=w245:refnum<class "A3200.lvclass">)  [unwired: 8 in, 1 out]
            n113 = Index Array(array=w244) -> (element #3=w242:dbl)  [unwired: 4 in, 3 out]
            n114 = Subtract(x=w242, y=10.0) -> (x-y=w241:dbl)
            n115 = call-dynamic "Z Go.vi"("Speed"=2.0, "Position"=w241, "Gantry in"=w245) -> ("Gantry out"=w247:refnum<class "A3200.lvclass">)  [unwired: 7 in, 1 out]
            n116 = call "XYZTheta Go.vi"("XYZTheta In"=w251, "Motion in"=w247) -> ("Motion out"=w250:refnum<class "A3200.lvclass">)  [unwired: 7 in, 2 out]
          }
          frame #2 {
            n117 = call "z go delay.vi"("Motion.lvclass"=w253) -> ("Motion.lvclass 2"=w252:refnum<class "A3200.lvclass">)  [unwired: 10 in]
            n118 = call "Lower_Stop.vi"("I-O in"=w256, "Motion in"=w252) -> ("I-O out"=w255:refnum<class "NI-DAQ.lvclass">, "Motion out"=w254:refnum<class "A3200.lvclass">)  [unwired: 7 in, 1 out]
          }
          frame #3 {
            n119 = call "IO sensor.vi"("Value"=FALSE, "Channel"=0, "I-O in"=w259) -> ("I-O out"=w258:refnum<class "NI-DAQ.lvclass">)  [unwired: 8 in]
          }
          frame #4 {
            n120 = call "XYZTheta Go.vi"("XYZTheta In"=w262, "Motion in"=w265) -> ("error out"=w263:errorcluster, "Motion out"=w264:refnum<class "A3200.lvclass">)  [unwired: 7 in, 1 out]
          }
        }
        n121 = call "Prompt User for Input"("error in (no error)"=w193) -> ("error out"=w192:errorcluster)  [unwired: 17 in, 1 out]
        n122 = call "Prompt User for Input3"("error in (no error)"=w202) -> ()  [unwired: 17 in, 2 out]
        n123 = Bundle By Name(cluster=w200, "A3200.lvclass"=w195, "NI-DAQ.lvclass"=w196) -> (w199:T4)
      }
      event "run 2": Value Change {
        n124 = event-data() -> ()  [unwired: 1 in, 6 out]
      }
      event "IO 1", "IO 2": Value Change {
        n125 = event-data() -> ()  [unwired: 1 in, 6 out]
        n126 = Unbundle By Name(w325) -> ("NI-DAQ.lvclass"=w324:refnum<class "NI-DAQ.lvclass">)
        n127 = case shown="True" "IO 1" {
          tunnel: w332 -> [_ w345]
          tunnel: w324 -> [w342 w343]
          tunnel: [w342 w344] -> w329
          frame False {
          }
          frame True {
            n128 = call-dynamic "Digital Write 1 Channel.vi"("Value"="Value", "Channel"=w345, "NI-DAQ.lvclass"=w343) -> ("NI-DAQ.lvclass 2"=w344:refnum<class "NI-DAQ.lvclass">)  [unwired: 7 in, 1 out]
          }
        }
        n129 = case shown="True" "IO 2" {
          tunnel: w331 -> [_ w341]
          tunnel: w330 -> [_ w340]
          tunnel: w329 -> [w337 w339]
          tunnel: [w337 w338] -> w326
          frame False {
          }
          frame True {
            n130 = call-dynamic "Digital Write Multiple Channels.vi"("Values"=w341, "Indices"=w340, "NI-DAQ in"=w339) -> ("NI-DAQ out"=w338:refnum<class "NI-DAQ.lvclass">)  [unwired: 7 in, 1 out]
          }
        }
        n131 = Bundle By Name(cluster=w325, "NI-DAQ.lvclass"=w326) -> (w327:T4)
      }
      event "go to Lower stop": Value Change {
        n132 = event-data() -> ()  [unwired: 1 in, 6 out]
        n133 = Unbundle By Name(w352) -> ("A3200.lvclass"=w348:refnum<class "A3200.lvclass">, "NI-DAQ.lvclass"=w351:refnum<class "NI-DAQ.lvclass">)
        n134 = call "Lower_Stop.vi"("I-O in"=w351, "Motion in"=w348) -> ("I-O out"=w350:refnum<class "NI-DAQ.lvclass">, "Motion out"=w349:refnum<class "A3200.lvclass">)  [unwired: 7 in, 1 out]
        n135 = Bundle By Name(cluster=w352, "A3200.lvclass"=w349, "NI-DAQ.lvclass"=w350) -> (w353:T4)
      }
      event "z to zero": Value Change {
        n136 = event-data() -> ()  [unwired: 1 in, 6 out]
        n137 = Unbundle By Name(w359) -> ("A3200.lvclass"=w358:refnum<class "A3200.lvclass">)
        n138 = call "Clear.vi"("Motion in"=w358) -> ("Motion out"=w360:refnum<class "A3200.lvclass">)  [unwired: 9 in, 1 out]
        n139 = Bundle By Name(cluster=w359, "A3200.lvclass"=w360) -> (w361:T4)
      }
      event "z go": Value Change {
        n140 = event-data() -> ()  [unwired: 1 in, 6 out]
        n141 = Unbundle By Name(w367) -> ("A3200.lvclass"=w368:refnum<class "A3200.lvclass">)
        n142 = call-dynamic "Z Go.vi"("Speed"=5.0, "Position"="Position", "Gantry in"=w368) -> ("Gantry out"=w365:refnum<class "A3200.lvclass">)  [unwired: 7 in, 1 out]
        n143 = Bundle By Name(cluster=w367, "A3200.lvclass"=w365) -> (w366:T4)
      }
    }
  }
  "controller out" <- w3
  "z offset out" <- w1
